vi "get fpga resources compatible with FPGA Addon CD group.vi"(8 "error in (no error)":errorcluster, 11 "Item Ref":T1 format="%.0x") -> (0 "error out":errorcluster, 3 "fpga resources":variant[](array[variant]))   [LabVIEW 2016, in "FPGA RM System Definition API.lvlib"]
doc: "Given a node pointer to Scalar Inputs, Scalar Outputs, Waveform Inputs, or Waveform Outputs, this reutrns all compatible FPGA resources associated with the parent FPGA Addon CD"
uses:
  FPGA-Resource-Manager-APIs/Source/System Definition/FPGA RM System Definition API.lvlib
  <vilib>/NI Veristand/Custom Device API/Custom Device Item Ref.ctl
  FPGA-Resource-Manager-APIs/Source/Channel Type.ctl
  <vilib>/NI VeriStand/Custom Device API/Custom Device API.lvlib
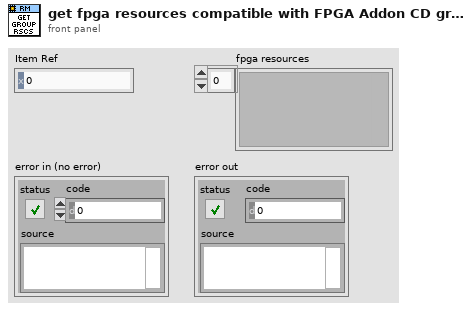
[diagram p1: front panel]
types:
  T1 = typedef "Custom Device API.lvlib/Custom Device Item Ref.ctl" = u64
  T2 = typedef "Custom Device API.lvlib/Custom Device Item Info.ctl" = cluster{"Name":string, "Is Channel":bool, "GUID":string, "Is Waveform":bool}
  T3 = typedef "FPGA RM System Definition API.lvlib/Channel Type.ctl" = enum16{"Write Channel", "Read Channel", "Write Waveform", "Read Waveform"}
  T4 = typedef "FPGA RM System Definition API.lvlib/fpga resource.ctl" = cluster{"name":string, "datatype":string, "channel type":T3, "value":variant, "notes":string}
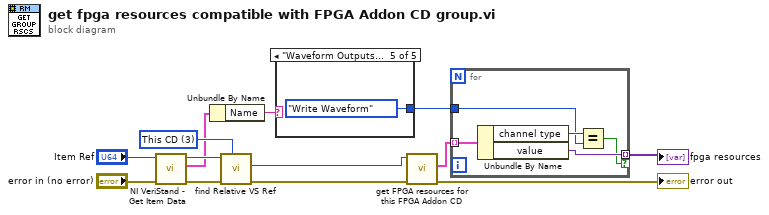
[diagram p0: block diagram]
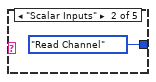
[diagram p3: hidden frame]
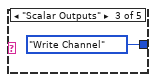
[diagram p4: hidden frame]
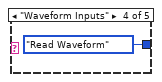
[diagram p5: hidden frame]
diagram:
  w7 = u16 3 items=["Targets", "Controller", "Custom Devices", "This CD", "This CD/Group", "This CD/Group/SubGroup"] ("Relative Type")
  n1 = call <vilib>:"NI VeriStand - Get Item Data.vi"("error in (no error)"="error in (no error)", "Item Ref in"="Item Ref") -> ("error out"=w5:errorcluster, "Item Info"=w3:T2, "Item Ref out"=w4:T1)  [unwired: 6 in, 1 out]
  n2 = Unbundle By Name(w3) -> ("Name"=w6:string)
  n3 = call "find Relative VS Ref.vi"("Relative Type"=w7, "error in (no error)"=w5, "Item Ref in"=w4) -> ("error out"=w9:errorcluster, "Relative Item Ref Out"=w8:T1)  [unwired: 4 in, 3 out]
  n4 = case shown="\"Waveform Outputs\"" w6 {
    tunnel: [_ Channel_Type."Read Channel" ("channel type") Channel_Type."Write Channel" ("y") Channel_Type."Read Waveform" ("y") Channel_Type."Write Waveform" ("y")] -> w13
    frame Default {
    }
    frame "Scalar Inputs" {
    }
    frame "Scalar Outputs" {
    }
    frame "Waveform Inputs" {
    }
    frame "Waveform Outputs" {
    }
  }
  n5 = call "get FPGA resources for this FPGA Addon CD.vi"("error in (no error)"=w9, "Item Ref in"=w8) -> ("error out"=→"error out":errorcluster, "fpga resources"=w10:T4[])  [unwired: 6 in, 2 out]
  n6 = for {
    tunnel: w10 -> [w22] mode=indexing
    tunnel: [w20] -> w11 mode=indexing if=w19
    tunnel: w13 -> [w18]
    n7 = Unbundle By Name(w22) -> ("channel type"=w21:T3, "value"=w20:variant)
    n8 = Equal?(x=w21, y=w18) -> (x = y?=w19:bool)
  }
  "fpga resources" <- w11
